vi "Shutter.vi"(8 "Error In":errorcluster, 11 "Simulate hardware?":bool) -> (0 "Error Out":errorcluster)   [LabVIEW 2017, in "Shutter.lvlib"]
uses:
  Shutter.lvlib
  Controls/Params.ctl
  Monochromator/Controls/VISA parameters.ctl
  Controls/Errors.ctl
  Events/Events.lvlib
  System Control/Main controller.lvlib
  Serial comms/Serial comms.lvlib
panel:
  in  "Shutter":T1={"Open command string"="+100\\s10\\n", "VISA"={"Timeout (ms)"=10000, "Resource Name"="COM1", "Baud Rate"=9600, "Data Bits"=8, "Parity"=0, "Stop Bits"=10, "Flow Control"=0}} {"VISA"."Flow Control" items=["None"=0, "XON/XOFF"=1, "RTS/CTS"=2, "DTR/DSR"=4]; "VISA"."Stop Bits" items=["1.0"=10, "1.5"=15, "2.0"=20]; "VISA"."Parity" items=["None", "Odd", "Even", "Mark", "Space"]}
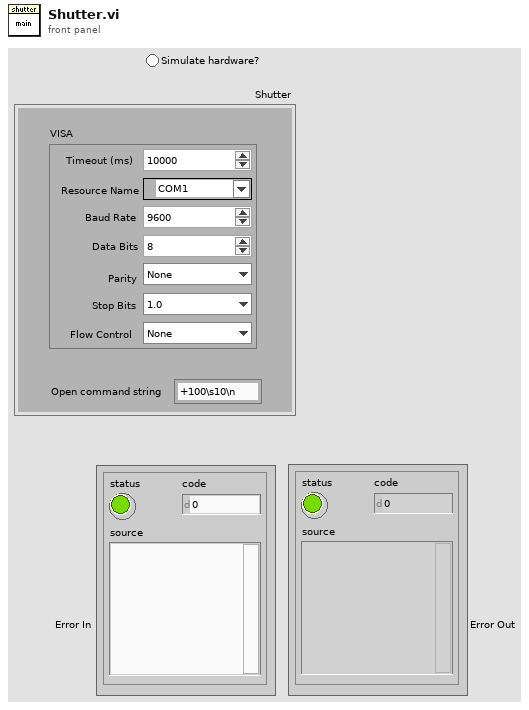
[diagram p1: front panel]
types:
  T1 = typedef "Shutter.lvlib/Params.ctl" = cluster{"Open command string":string, "VISA":T2}
  T2 = typedef "Serial comms.lvlib/VISA parameters.ctl" = cluster{"Timeout (ms)":u32, "Resource Name":refnum<visa-resource-name>, "Baud Rate":u32, "Data Bits":u16, "Parity":u16, "Stop Bits":u16, "Flow Control":u16}
  T3 = typedef "Events.lvlib/Refs [cluster].ctl" = cluster{"Exit":refnum<user-event>, "Controller":refnum<user-event>, "System Error":refnum<user-event>, "UI":refnum<user-event>, "Example Module":refnum<user-event>, "Shutter":refnum<user-event>, "Monochromator":refnum<user-event>, "DAQ":refnum<user-event>, "Scope":refnum<user-event>, "Processing":refnum<user-event>, "File IO":refnum<user-event>, "Colour wheel":refnum<user-event>}
  T4 = typedef "Shutter.lvlib/Errors.ctl" = cluster{"Bad wait time":errorcluster}
  T5 = typedef "Shutter.lvlib/Module Commands [enum].ctl" = enum16{"Start", "Move", "Return", "Stop"}
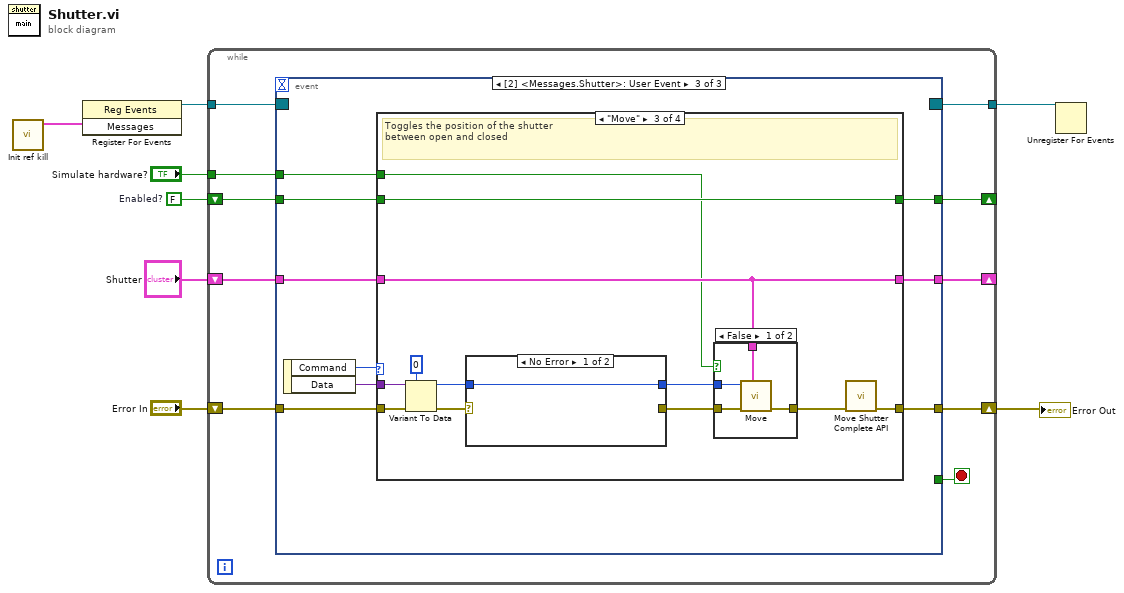
[diagram p0: block diagram]
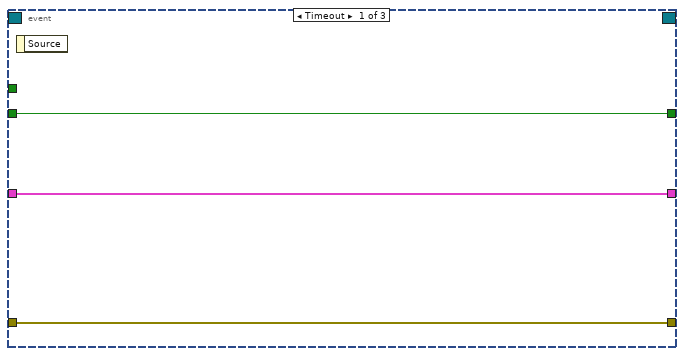
[diagram p2: hidden frame]
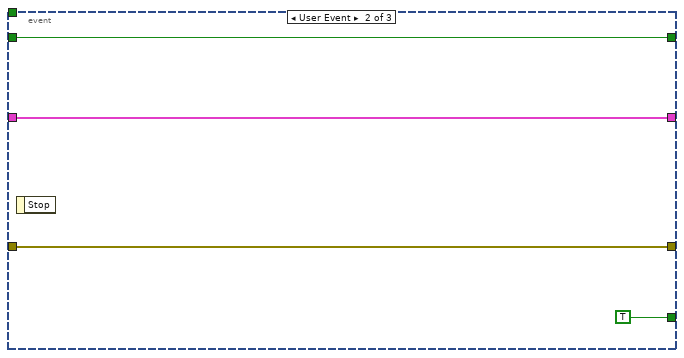
[diagram p3: hidden frame]
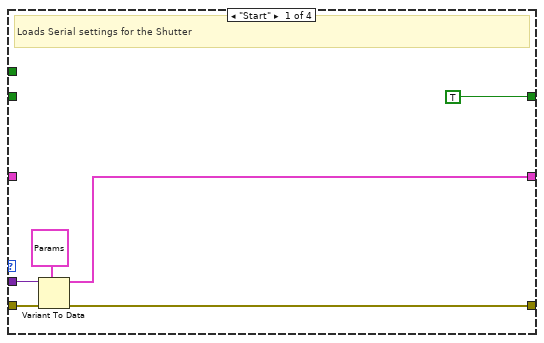
[diagram p4: hidden frame]
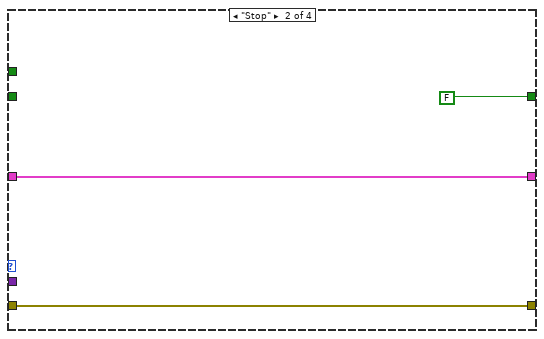
[diagram p5: hidden frame]
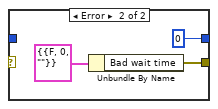
[diagram p7: hidden frame]
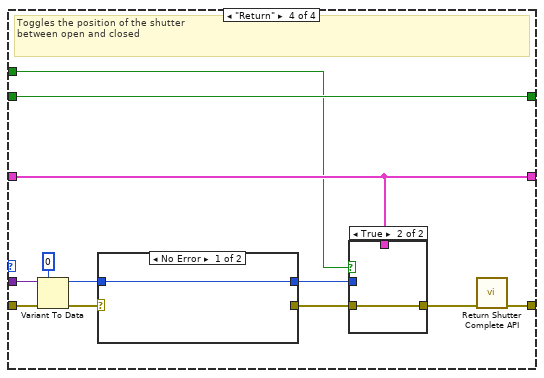
[diagram p8: hidden frame]
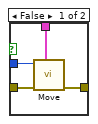
[diagram p9: hidden frame]
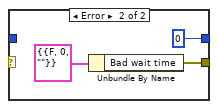
[diagram p10: hidden frame]
diagram:
  w6 = FALSE  # Enabled?
  n1 = call "Init ref kill.vi"() -> ("Messages"=w8:T3)  [unwired: 10 in, 1 out]
  n2 = register-events(w8) -> (reference out=w7:refnum<event-registration>)  [unwired: 2 in, 1 out]
  n3 = while {
    tunnel: w7 -> [w18]
    shift-right: [w15] -> _
    shift-left: w6 -> [w14]
    tunnel: [w16] -> w5
    shift-right: [w12] -> w3
    shift-left: "Error In" -> [w13]
    shift-right: [w10] -> _
    shift-left: "Shutter" -> [w11]
    tunnel: "Simulate hardware?" -> [w9]
    stop <- w17 stop-if-true
    n4 = event shown="[2] <Messages.Shutter>: User Event" {
      selector: w18 -> [_ _ _]
      dyn-events: [_ _ _] -> w16
      timeout: _ -> [_ _ _]
      tunnel: [_ TRUE _] -> w17
      tunnel: [w21 w22 w33] -> w15
      tunnel: w14 -> [w21 w22 w32]
      tunnel: w13 -> [w19 w23 w30]
      tunnel: [w19 w23 w29] -> w12
      tunnel: w11 -> [w20 w24 w28]
      tunnel: [w20 w24 w27] -> w10
      tunnel: w9 -> [_ _ w26]
      event Timeout {
        n5 = event-data() -> ()  [unwired: 1 in, 1 out]
      }
      event User Event {
        n6 = event-data() -> ()  [unwired: 1 in, 1 out]
      }
      event User Event {
        n7 = event-data() -> ("Command"=w34:T5, "Data"=w31:variant)  [unwired: 1 in]
        n8 = case shown="\"Move\"" w34 {
          tunnel: [TRUE FALSE w55 w76] -> w33
          tunnel: w32 -> [_ _ w55 w76]
          tunnel: w31 -> [w39 _ w54 w75]
          tunnel: w30 -> [w38 w41 w52 w73]
          tunnel: [w35 w41 w46 w66] -> w29
          tunnel: w28 -> [_ w42 w51 w72]
          tunnel: [w36 w42 w51 w72] -> w27
          tunnel: w26 -> [_ _ w44 w65]
          frame "Start" {
            # "Loads Serial settings for the Shutter"
            n9 = Variant To Data(error in=w38, type=T1 {"Open command string"="+100\\s10\\n", "VISA"={"Timeout (ms)"=10000, "Resource Name"="COM1", "Baud Rate"=9600, "Data Bits"=8, "Parity"=0, "Stop Bits"=10, "Flow Control"=0}} ("Shutter"), Variant=w39) -> (data=w36:T1, error out=w35:errorcluster)
          }
          frame "Stop" {
          }
          frame "Move" {
            # "Toggles the position of the shutter \nbetween open and closed"
            n10 = Variant To Data(error in=w52, type=u32 0, Variant=w54) -> (data=w48:u32, error out=w50:errorcluster)
            n11 = case shown="No Error" w50 {
              tunnel: [_ w62] -> w49
              tunnel: w48 -> [w61 _]
              tunnel: [w61 u32 0] -> w47
              frame No Error {
              }
              frame Error {
                n12 = Unbundle By Name(T4 {"Bad wait time"={"status"=FALSE, "code"=0, "source"=""}} ("Errors")) -> ("Bad wait time"=w62:errorcluster)
              }
            }
            n13 = case shown="False" w44 {
              tunnel: w51 -> [w59 _]
              tunnel: w49 -> [w58 w60]
              tunnel: w47 -> [w57 _]
              tunnel: [w56 w60] -> w45
              frame False {
                n14 = call "Move.vi"("Shutter"=w59, "error in (no error)"=w58, "milliseconds to wait"=w57) -> ("error out"=w56:errorcluster)  [unwired: 8 in]
              }
              frame True {
              }
            }
            n15 = call "Move Shutter Complete API.vi"("Error In"=w45) -> ("Error Out"=w46:errorcluster)  [unwired: 10 in]
          }
          frame "Return" {
            # "Toggles the position of the shutter \nbetween open and closed"
            n16 = Variant To Data(error in=w73, type=u32 0, Variant=w75) -> (data=w69:u32, error out=w71:errorcluster)
            n17 = case shown="No Error" w71 {
              tunnel: [_ w83] -> w70
              tunnel: w69 -> [w82 _]
              tunnel: [w82 u32 0] -> w68
              frame No Error {
              }
              frame Error {
                n18 = Unbundle By Name(T4 {"Bad wait time"={"status"=FALSE, "code"=0, "source"=""}} ("Errors")) -> ("Bad wait time"=w83:errorcluster)
              }
            }
            n19 = case shown="True" w65 {
              tunnel: w72 -> [w80 _]
              tunnel: w70 -> [w79 w81]
              tunnel: w68 -> [w78 _]
              tunnel: [w77 w81] -> w67
              frame False {
                n20 = call "Move.vi"("Shutter"=w80, "error in (no error)"=w79, "milliseconds to wait"=w78) -> ("error out"=w77:errorcluster)  [unwired: 8 in]
              }
              frame True {
              }
            }
            n21 = call "Return Shutter Complete API.vi"("Error In"=w67) -> ("Error Out"=w66:errorcluster)  [unwired: 10 in]
          }
        }
      }
    }
  }
  "Error Out" <- w3
  n22 = Unregister For Events(event registration refnum=w5) -> ()  [unwired: 1 in, 1 out]
